vi "Loop.vi"(11 "Hello World Event in":refnum<class "Hello World Event.lvclass">) -> (3 "Hello World Event out":refnum<class "Hello World Event.lvclass">)   [LabVIEW 2021, in "Hello World Event.lvlib" / "Hello World Event.lvclass"]
uses:
  Hello World Event.lvclass
  Hello World Event.lvclass/Hello World Event.ctl
  Hello World Queue/Hello World Queue/Hello World Queue.lvclass
  jettl Msg Teardown/jettl Msg Teardown.lvlib
  jettl Msg Queue Create/jettl Msg Queue Create.lvlib
  jettl/Event jettl/Event jettl.lvclass
  jettl/Msg Strategy/Msg Strategy.lvclass
  jettl Msg String Indicator/jettl Msg String Indicator.lvlib
  jettl Msg Pop Up/jettl Msg Pop Up.lvlib
  C:/git/jettl/src/jettl/jettl/jettl.lvclass
  C:/git/jettl/src/jettl Msg Merge Error/Merge Error/Merge Error.lvclass
  C:/git/jettl/src/jettl/Event jettl/Event jettl.lvclass
  C:/git/jettl/src/jettl Msg Override Error/Override Error/Override Error.lvclass
  C:/git/jettl/src/jettl Msg Setup/Setup/Setup.lvclass
  C:/git/jettl/src/jettl Msg Teardown/Teardown/Teardown.lvclass
  C:/git/jettl/src/Hello World/Hello World Event/Hello World Event/Hello World Event.lvclass
  C:/git/jettl/src/Hello World/jettl Msg String Indicator/String Indicator/String Indicator.lvclass
  jettl Msg Pop Up/Pop Up Msg Strategy/Pop Up Msg Strategy.lvclass
  C:/git/jettl/src/Hello World/jettl Msg Pop Up/Pop Up Msg Strategy/Pop Up Msg Strategy.lvclass
  C:/git/jettl/src/jettl/Msg Strategy/Msg Strategy.lvclass
  jettl Msg Teardown/Teardown Msg Strategy/Teardown Msg Strategy.lvclass
  C:/git/jettl/src/jettl Msg Teardown/Teardown Msg Strategy/Teardown Msg Strategy.lvclass
  C:/git/jettl/src/jettl/Queue jettl/Queue jettl.lvclass
  C:/git/jettl/src/jettl Msg Event Create/Event Create/Event Create.lvclass
  C:/git/jettl/src/jettl Msg Queue Create/Queue Create/Queue Create.lvclass
  C:/git/jettl/src/jettl/jettl Msg Event Last Ack/Event Last Ack/Event Last Ack.lvclass
  C:/git/jettl/src/jettl/jettl Msg Queue Last Ack/Queue Last Ack/Queue Last Ack.lvclass
  C:/git/jettl/src/Hello World/Hello World Queue/Hello World Queue/Hello World Queue.lvclass
  C:/git/jettl/src/Hello World/jettl Msg Pop Up/Pop Up/Pop Up.lvclass
  jettl Msg Queue Create/Queue Create Msg Strategy/Queue Create Msg Strategy.lvclass
  C:/git/jettl/src/jettl Msg Queue Create/Queue Create Msg Strategy/Queue Create Msg Strategy.lvclass
  jettl Msg String Indicator/String Indicator Msg Strategy/String Indicator Msg Strategy.lvclass
  C:/git/jettl/src/Hello World/jettl Msg String Indicator/String Indicator Msg Strategy/String Indicator Msg Strategy.lvclass
panel:
  in  "Nested Name":string
  in  "Create Nested":bool
  out "String Indicator":string
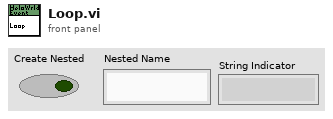
[diagram p1: front panel]
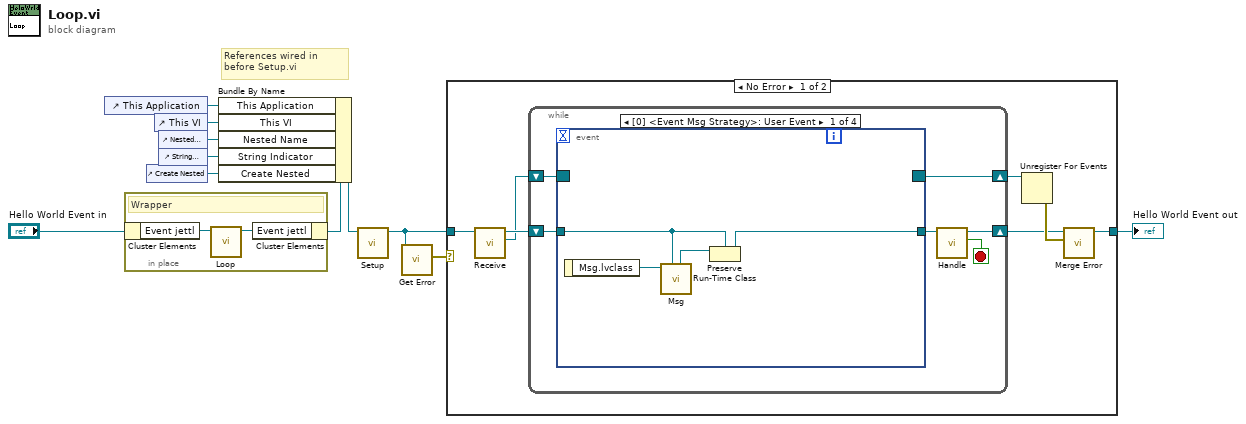
[diagram p0: block diagram]
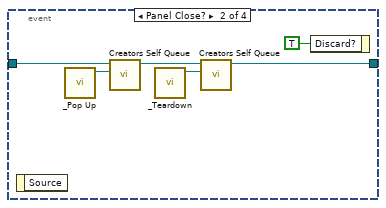
[diagram p2: hidden frame]
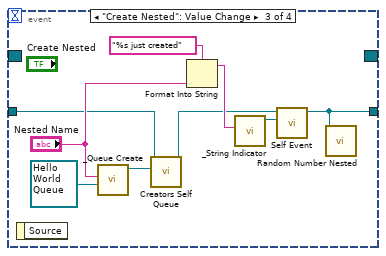
[diagram p3: hidden frame]
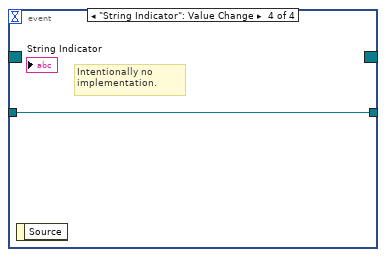
[diagram p4: hidden frame]
diagram:
  # "References wired in before Setup.vi"
  n1 = control-ref of="This Application"() -> (w2:refnum<vi>)
  n2 = in-place {
    # "Wrapper"
    n3 = in-place-cluster #1("Hello World Event in") -> ("Event jettl"=w13:refnum<class "Event jettl.lvclass">)
    n4 = call-dynamic "Loop.vi"("Event jettl in"=w13) -> ("Event jettl out"=w12:refnum<class "Event jettl.lvclass">)  [unwired: 10 in]
    n5 = in-place-cluster #1("Event jettl"=w12) -> (w11:refnum<class "Hello World Event.lvclass">)
  }
  n6 = control-ref of="Create Nested"() -> (w1:refnum<vi>)
  n7 = control-ref of="This VI"() -> (w10:refnum<vi>)
  n8 = control-ref of="Nested Name"() -> (w7:refnum<vi>)
  n9 = control-ref of="String Indicator"() -> (w3:refnum<vi>)
  n10 = Bundle By Name(cluster=w11, "This Application"=w2, "This VI"=w10, "Nested Name"=w7, "String Indicator"=w3, "Create Nested"=w1) -> (w6:refnum<class "Hello World Event.lvclass">)
  n11 = call-dynamic "Setup.vi"("Hello World Event in"=w6) -> ("Hello World Event out"=w4:refnum<class "Hello World Event.lvclass">)  [unwired: 10 in]
  n12 = call-dynamic "Get Error.vi"("Hello World Event in"=w4) -> ("Error"=w5:errorcluster)  [unwired: 10 in]
  n13 = case shown="No Error" w5 {
    tunnel: [w19 w47] -> w9
    tunnel: w4 -> [w17 w47]
    frame No Error {
      n14 = call-dynamic "Receive.vi"("Hello World Event in"=w17) -> ("Registration"=w15:refnum<event-registration>, "Hello World Event out"=w18:refnum<class "Hello World Event.lvclass">)  [unwired: 9 in]
      n15 = while {
        shift-right: [w25] -> w14
        shift-left: w18 -> [w21]
        shift-right: [w22] -> w20
        shift-left: w15 -> [w26]
        stop <- w24 stop-if-true
        n16 = event "UI Events" shown="[0] <Event Msg Strategy>: User Event" {
          selector: w26 -> [_ _ _ _]
          dyn-events: [_ _ _ _] -> w22
          timeout: _ -> [_ _ _ _]
          tunnel: [w27 w35 w38 w46] -> w23
          tunnel: w21 -> [w28 w33 w40 w46]
          event User Event {
            n17 = event-data() -> ("Msg.lvclass"=w29:refnum<class "Msg Strategy.lvclass">)  [unwired: 1 in]
            n18 = call-dynamic "Msg.vi"("jettl in"=w28, "Msg Strategy in"=w29) -> ("jettl out"=w30:refnum<class "jettl.lvclass">)  [unwired: 9 in]
            n19 = Preserve Run-Time Class(object in=w30, 2:w28) -> (object out=w27:refnum<class "Hello World Event.lvclass">)  [unwired: 1 in, 1 out]
          }
          event Panel Close? {
            n20 = event-data() -> ()  [unwired: 1 in, 1 out]
            n21 = call "_Pop Up.vi"() -> ("Pop Up Msg Strategy out"=w31:refnum<class "Pop Up Msg Strategy.lvclass">)  [unwired: 11 in]
            n22 = call-dynamic "Creators Self Queue.vi"("Msg Strategy"=w31, "Hello World Event in"=w33) -> ("Hello World Event out"=w32:refnum<class "Hello World Event.lvclass">)  [unwired: 9 in]
            n23 = call "_Teardown.vi"() -> ("Teardown Msg Strategy out"=w34:refnum<class "Teardown Msg Strategy.lvclass">)  [unwired: 11 in]
            n24 = call-dynamic "Creators Self Queue.vi"("Msg Strategy"=w34, "Hello World Event in"=w32) -> ("Hello World Event out"=w35:refnum<class "Hello World Event.lvclass">)  [unwired: 9 in]
            n25 = event-data("Discard?"=TRUE) -> ()  [unwired: 1 in, 1 out]
          }
          event "Create Nested": Value Change {
            n26 = event-data() -> ()  [unwired: 1 in, 1 out]
            n27 = call "_Queue Create.vi"("Queue jettl"=refnum<class "Hello World Queue.lvclass"> refnum ("Hello World Queue.lvlib:Hello World Queue.lvclass"), "Alias"="Nested Name") -> ("Queue Create Msg Strategy out"=w41:refnum<class "Queue Create Msg Strategy.lvclass">)  [unwired: 9 in]
            n28 = call-dynamic "Creators Self Queue.vi"("Msg Strategy"=w41, "Hello World Event in"=w40) -> ("Hello World Event out"=w39:refnum<class "Hello World Event.lvclass">)  [unwired: 9 in]
            n29 = Format Into String(format string="%s just created", "Nested Name") -> (resulting string=w42:string)  [unwired: 2 in, 1 out]
            n30 = call "_String Indicator.vi"("String Indicator"=w42) -> ("String Indicator Msg Strategy out"=w37:refnum<class "String Indicator Msg Strategy.lvclass">)  [unwired: 10 in]
            n31 = call-dynamic "Self Event.vi"("Msg Strategy"=w37, "Hello World Event in"=w39) -> ("Hello World Event out"=w38:refnum<class "Hello World Event.lvclass">)  [unwired: 9 in]
            n32 = call "Random Number Nested.vi"("Hello World Event in"=w38) -> ()  [unwired: 11 in]
          }
          event "String Indicator": Value Change {
            # "Intentionally no implementation."
            n33 = event-data() -> ()  [unwired: 1 in, 1 out]
          }
        }
        n34 = call-dynamic "Handle.vi"("Hello World Event in"=w23) -> ("Destroy?"=w24:bool, "Hello World Event out"=w25:refnum<class "Hello World Event.lvclass">)  [unwired: 9 in]
      }
      n35 = Unregister For Events(event registration refnum=w20) -> (error out=w16:errorcluster)  [unwired: 1 in]
      n36 = call-dynamic "Merge Error.vi"("Error"=w16, "Hello World Event in"=w14) -> ("Hello World Event out"=w19:refnum<class "Hello World Event.lvclass">)  [unwired: 9 in]
    }
    frame Error {
    }
  }
  "Hello World Event out" <- w9
